vi "Process UDP Output.vi"(0 "UDP Network Connection in":refnum<k16>, 1 "Data From Xplane":sgl[](array[numeric]), 3 "IP Address":u32, 4 "Port":i32, 5 "error in (no error)":errorcluster, 6 "Elevator":sgl, 8 "Aileron":sgl, 10 "Rudder":sgl, 12 "Throttle":sgl) -> (14 "UDP Network \nConnection out":refnum<k16>, 19 "error out":errorcluster)   [LabVIEW 2014]
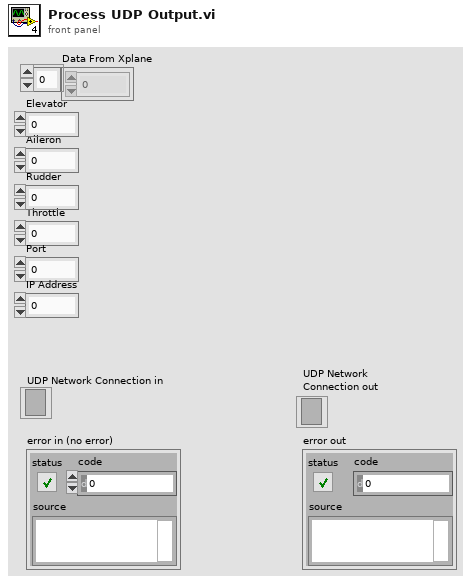
[diagram p1: front panel]
types:
  T1 = enum16{"big-endian, network order", "native, host order", "little-endian"}
  T2 = cluster{"[0]":sgl, "[1]":sgl, "[2]":sgl, "[3]":sgl, "[4]":sgl, "[5]":sgl, "[6]":sgl, "[7]":sgl, "[8]":sgl}
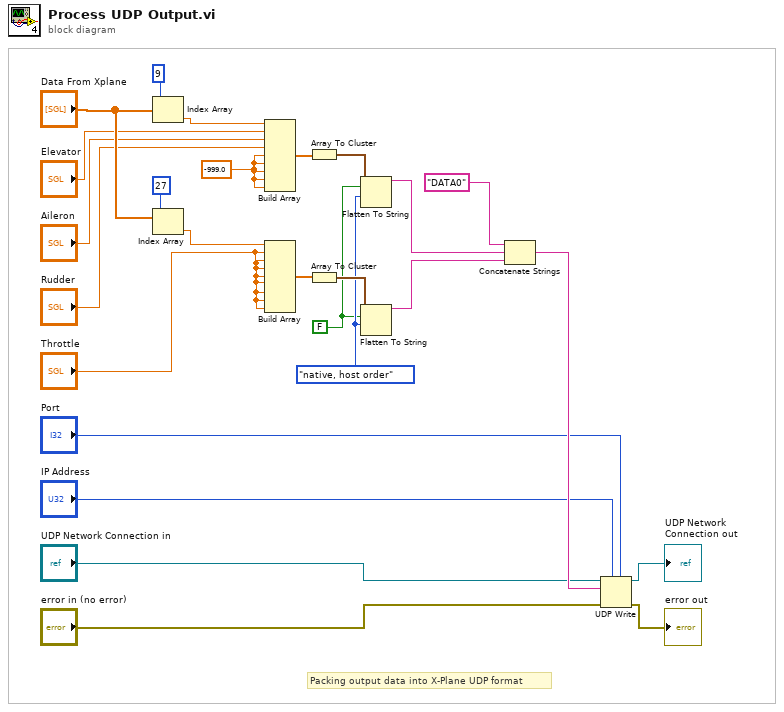
[diagram p0: block diagram]
diagram:
  w3 = T1."native, host order" ("byte order (0:big-endian, network order)")
  w2 = FALSE ("prepend array or string size? (T)")
  w12 = sgl -999.0 ("element")
  # "Packing output data into X-Plane UDP format"
  n1 = Index Array(array="Data From Xplane", index=9) -> (element=w11:sgl)
  n2 = Index Array(array="Data From Xplane", index=27) -> (element=w22:sgl)
  n3 = Build Array(w11, "Elevator", "Aileron", "Rudder", w12, w12, w12, w12, w12) -> (w16:sgl[])
  n4 = Build Array(w22, "Throttle", "Throttle", "Throttle", "Throttle", "Throttle", "Throttle", "Throttle", "Throttle") -> (w23:sgl[])
  n5 = Array To Cluster(array=w16) -> (cluster=w17:T2)
  n6 = Array To Cluster(array=w23) -> (cluster=w24:T2)
  n7 = Flatten To String(anything=w17, prepend array or string size? (T)=w2, byte order (0:big-endian, network order)=w3) -> (data string=w14:string)  [unwired: 1 in, 2 out]
  n8 = Flatten To String(anything=w24, prepend array or string size? (T)=w2, byte order (0:big-endian, network order)=w3) -> (data string=w25:string)  [unwired: 1 in, 2 out]
  n9 = Concatenate Strings("DATA0", w14, w25) -> (w15:string)
  n10 = UDP Write(address="IP Address", port or service name="Port", connection ID="UDP Network Connection in", data in=w15, 8:"error in (no error)") -> (error out=→"error out":errorcluster, 3:→"UDP Network \nConnection out":refnum<k16>)  [unwired: 1 in]
